vi "ExposeBindControl.vi"(8 "Binding Type":T1=enum."Bidrectional", 9 "Controls":refnum<vi>[](array[refnum]), 10 "Control":refnum<vi>, 11 "Expose Info":T2) -> ()   [LabVIEW 2017]
uses:
  Core/ExposeInfo.ctl
  C:/Code/CMCryoSysCode/Expose/COM/CSCom/CSCom/bin/Release/CSCom.dll
  COM/CSCom/CSCom/bin/Release/CSCom.dll
  ExposeParameterBindingType.ctl
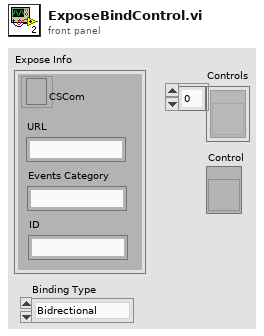
[diagram p1: front panel]
types:
  T1 = typedef "ExposeParameterBindingType.ctl" = enum16{"ToRemote", "FromRemote", "Bidrectional"}
  T2 = typedef "ExposeInfo.ctl" = cluster{"CSCom":refnum<k24>, "URL":string, "Events Category":string, "ID":string}
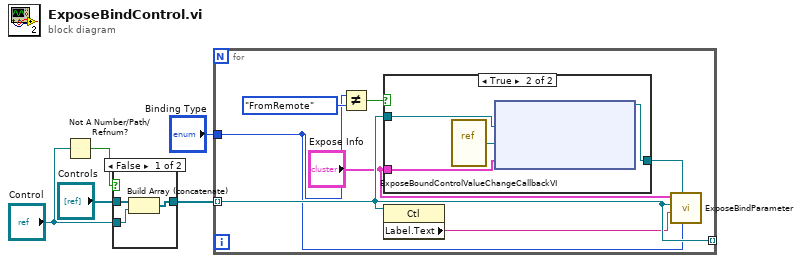
[diagram p0: block diagram]
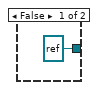
[diagram p2: hidden frame]
diagram:
  n1 = Not A Number/Path/Refnum?(number/path/refnum="Control") -> (NaN/Path/Refnum?=w5:bool)
  n2 = case shown="False" w5 {
    tunnel: "Controls" -> [w8 w9]
    tunnel: [w6 w9] -> w2
    tunnel: "Control" -> [w7 _]
    frame False {
      n3 = Build Array (concatenate)(w8, w7) -> (w6:refnum<vi>[])
    }
    frame True {
    }
  }
  n4 = for {
    tunnel: w2 -> [w14] mode=indexing
    tunnel: [w14] -> _ mode=indexing
    tunnel: "Binding Type" -> [w10]
    n5 = Not Equal?(x=w10, y=ExposeParameterBindingType."FromRemote") -> (x != y?=w15:bool)
    n6 = case shown="True" w15 {
      tunnel: w14 -> [_ w21]
      tunnel: [refnum<k27> refnum ("Event Callback") w20] -> w11
      tunnel: "Expose Info" -> [_ w19]
      frame False {
      }
      frame True {
        n7 = vi-ref "ExposeBoundControlValueChangeCallbackVI.vi"() -> ("vi reference"=w18:refnum<vi>)
        n8 = node(w21, w18, w19) -> (w20:refnum<k27>)  [unwired: 2 in, 1 out]
      }
    }
    n9 = property class="Ctl"(reference=w14) -> ("Label.Text"=w13:string)  [unwired: 1 in, 2 out]
    n10 = call "ExposeBindParameter.vi"("Bind Direction"=w10, "Val Change EV"=w11, "Name (empty)"=w13, "Value"=w14, "Expose Info"="Expose Info") -> ()  [unwired: 7 in]
  }
